vi "Config.vi"(1 "Config_W/R":bool, 2 "Config":T1={"IP"="192.168.0.1", "UserName"="admin", "Password"="admin", "boards_selector_group 1"=0, "boards_selector_group 2"=0, "log_name_group1"="G1", "log_name_group2"="G2", "Port"="COM5", "Delay[s]"=1.0, "on/off"=TRUE, "Graphs_color"=16448250, "Pages_color"=[6901059, 10986955, 11240591, 32639, 32639, 32639, 32639, 16777224, 9868950, 4417895, 8686180, 8686180, 8686180, 8686180], "logs_Path"=path "C:/Users/NEOVP/Documents/HV_DATA"} {"Delay[s]" format="%#_13g"}) -> (0 "Config_read":T1={"IP"="192.168.0.1", "UserName"="admin", "Password"="admin", "boards_selector_group 1"=0, "boards_selector_group 2"=0, "log_name_group1"="G1", "log_name_group2"="G2", "Port"="", "Delay[s]"=1.0, "on/off"=TRUE, "Graphs_color"=16448250, "Pages_color"=[6901059, 10986955, 11240591, 32639, 32639, 32639, 32639, 16777224, 9868950, 4417895, 8686180, 8686180, 8686180, 8686180], "logs_Path"=path ""} {"Delay[s]" format="%#_13g"})   [LabVIEW 2018]
uses:
  <vilib>/Utility/config.llb/Read Key (String).vi
  <vilib>/Utility/config.llb/Read Key (I32).vi
  <vilib>/Utility/config.llb/Read Key (Path).vi
  <vilib>/Utility/config.llb/Read Key (Double).vi
  <vilib>/Utility/config.llb/Read Key (Boolean).vi
  <vilib>/Utility/config.llb/Write Key (String).vi
  <vilib>/Utility/config.llb/Write Key (I32).vi
  <vilib>/Utility/config.llb/Write Key (Path).vi
  <vilib>/Utility/config.llb/Write Key (Double).vi
  <vilib>/Utility/config.llb/Write Key (Boolean).vi
  <vilib>/Utility/config.llb/NI_LVConfig.lvlib
panel:
  in  "Config Template":T1={"IP"="192.168.0.1", "UserName"="admin", "Password"="admin", "boards_selector_group 1"=0, "boards_selector_group 2"=0, "log_name_group1"="G1", "log_name_group2"="G2", "Port"="COM5", "Delay[s]"=1.0, "on/off"=TRUE, "Graphs_color"=16448250, "Pages_color"=[6901059, 10986955, 11240591, 32639, 32639, 32639, 32639, 16777224, 9868950, 4417895, 8686180, 8686180, 8686180, 8686180], "logs_Path"=path "C:/Users/NEOVP/Documents/HV_DATA"} {"Delay[s]" format="%#_13g"}
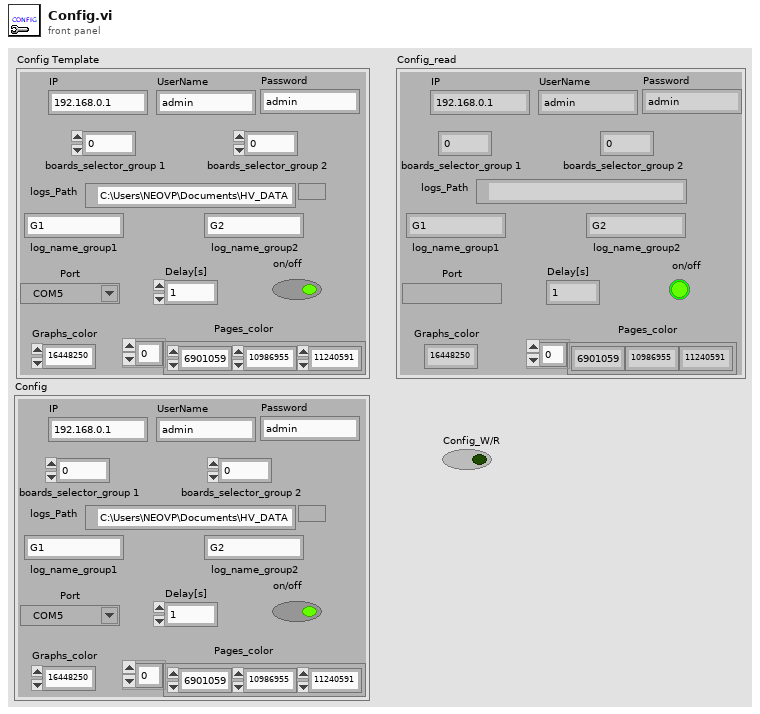
[diagram p1: front panel]
types:
  T1 = cluster{"IP":string, "UserName":string, "Password":string, "boards_selector_group 1":i32, "boards_selector_group 2":i32, "log_name_group1":string, "log_name_group2":string, "Port":refnum<visa-resource-name>, "Delay[s]":dbl, "on/off":bool, "Graphs_color":i32, "Pages_color":i64[], "logs_Path":path}
  T2 = typedef "NI_LVConfig.lvlib/Config Data RefNum.ctl" = refnum<k1>
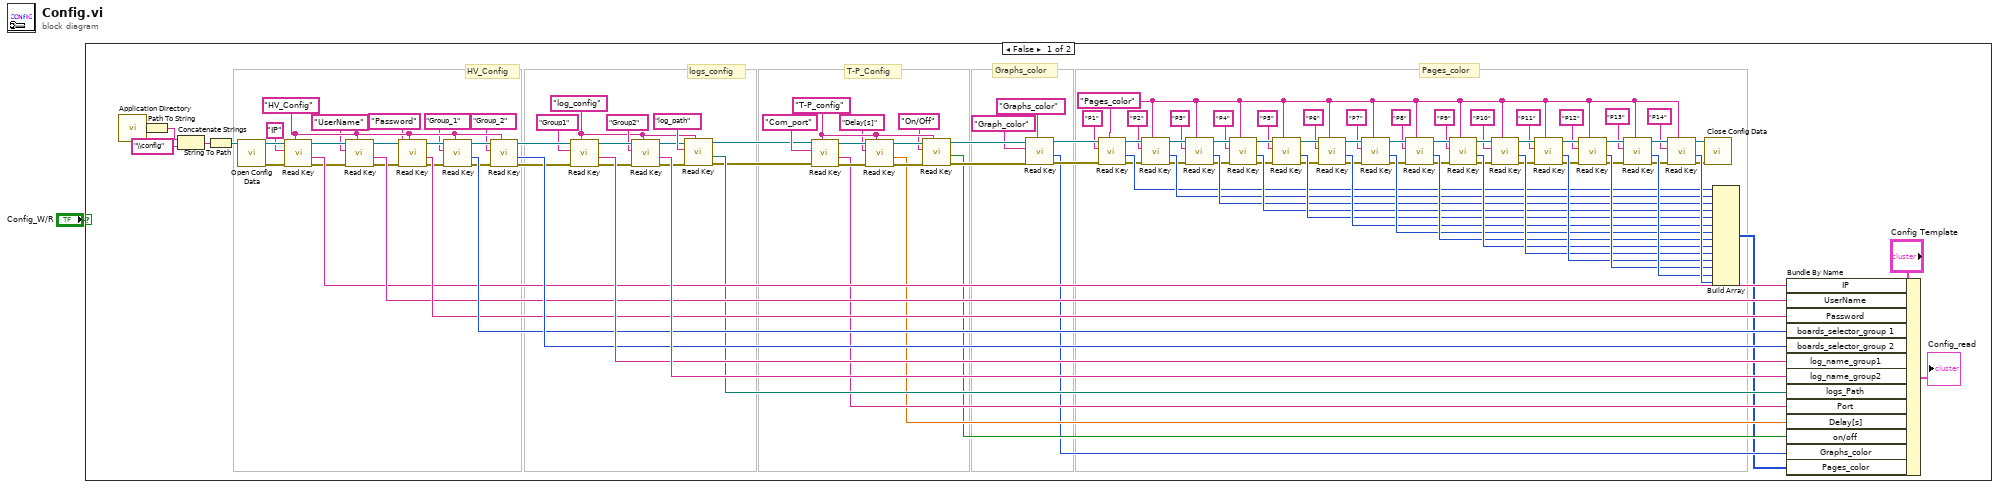
[diagram p0: block diagram]
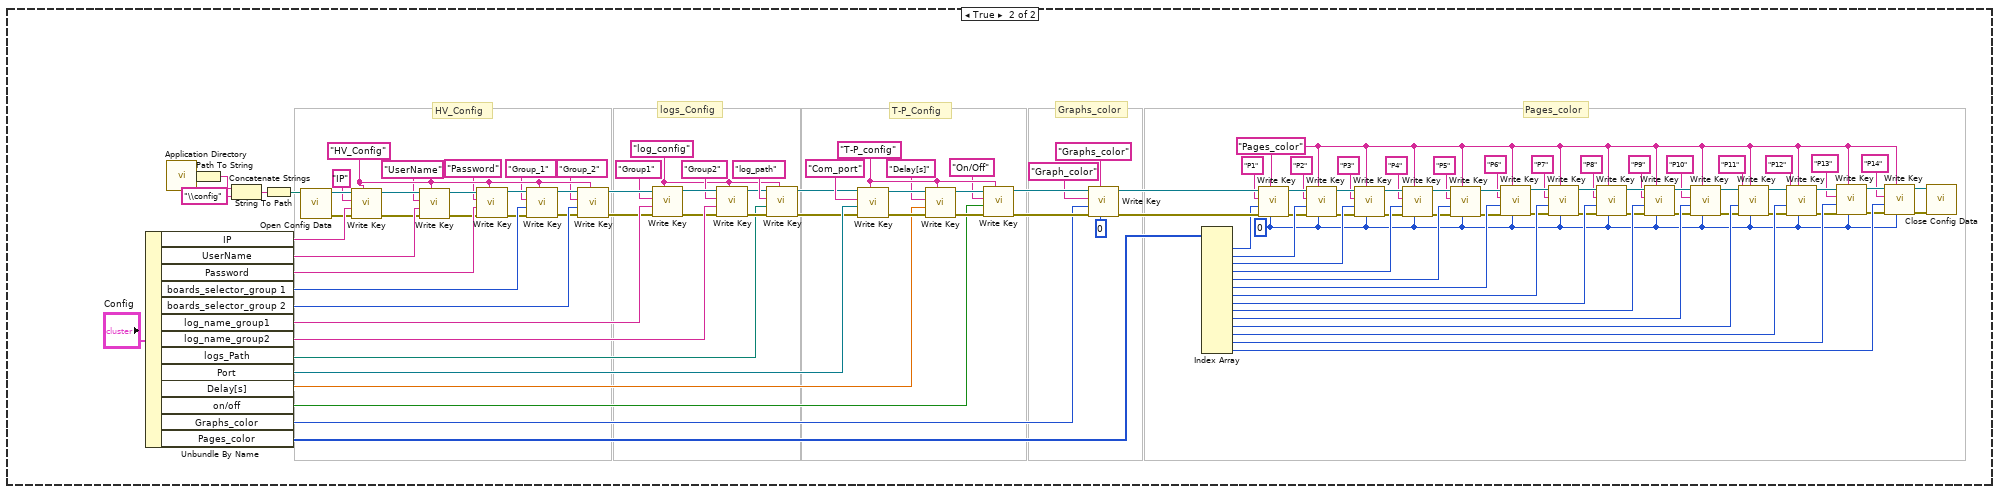
[diagram p2: hidden frame]
diagram:
  n1 = case shown="False" "Config_W/R" {
    frame False {
      w12 = "log_config" ("section")
      w41 = "HV_Config" ("section")
      w35 = "T-P_config" ("section")
      w29 = "Pages_color" ("section")
      # "logs_config"
      # "Pages_color"
      # "Graphs_color"
      # "T-P_Config"
      # "HV_Config"
      n2 = call <vilib>:"Application Directory.vi"() -> ("Application Directory"=w46:path)
      n3 = Path To String(path=w46) -> (string=w45:string)
      n4 = Concatenate Strings(w45, "\\config" ("string")) -> (w44:string)
      n5 = String To Path(string=w44) -> (path=w107:path)
      n6 = call <vilib>:"Open Config Data.vi"("configuration file path"=w107) -> ("error out"=w105:errorcluster, "refnum"=w106:T2)  [unwired: 8 in, 1 out]
      n7 = call-poly <vilib>:"Read Key.vi"("section"=w41, "error in (no error)"=w105, "key"="IP", "refnum"=w106) -> ("error out"=w103:errorcluster, "value"=w110:string, "refnum out"=w104:T2)  [unwired: 4 in, 1 out]
      n8 = call-poly <vilib>:"Read Key.vi"("section"=w41, "error in (no error)"=w103, "key"="UserName", "refnum"=w104) -> ("error out"=w101:errorcluster, "value"=w111:string, "refnum out"=w102:T2)  [unwired: 4 in, 1 out]
      n9 = call-poly <vilib>:"Read Key.vi"("section"=w41, "error in (no error)"=w101, "key"="Password", "refnum"=w102) -> ("error out"=w99:errorcluster, "value"=w112:string, "refnum out"=w100:T2)  [unwired: 4 in, 1 out]
      n10 = call-poly <vilib>:"Read Key.vi"("section"=w41, "error in (no error)"=w99, "key"="Group_1", "refnum"=w100) -> ("error out"=w97:errorcluster, "value"=w113:i32, "refnum out"=w98:T2)  [unwired: 4 in, 1 out]
      n11 = call-poly <vilib>:"Read Key.vi"("section"=w41, "error in (no error)"=w97, "key"="Group_2", "refnum"=w98) -> ("error out"=w93:errorcluster, "value"=w114:i32, "refnum out"=w94:T2)  [unwired: 4 in, 1 out]
      n12 = call-poly <vilib>:"Read Key.vi"("section"=w12, "error in (no error)"=w93, "key"="Group1", "refnum"=w94) -> ("error out"=w96:errorcluster, "value"=w115:string, "refnum out"=w95:T2)  [unwired: 4 in, 1 out]
      n13 = call-poly <vilib>:"Read Key.vi"("section"=w12, "error in (no error)"=w96, "key"="Group2", "refnum"=w95) -> ("error out"=w3:errorcluster, "value"=w116:string, "refnum out"=w5:T2)  [unwired: 4 in, 1 out]
      n14 = call-poly <vilib>:"Read Key.vi"("section"=w12, "error in (no error)"=w3, "key"="log_path", "refnum"=w5) -> ("error out"=w2:errorcluster, "value"=w11:path, "refnum out"=w4:T2)  [unwired: 4 in, 1 out]
      n15 = call-poly <vilib>:"Read Key.vi"("section"=w35, "error in (no error)"=w2, "key"="Com_port", "refnum"=w4) -> ("error out"=w90:errorcluster, "value"=w10:string, "refnum out"=w89:T2)  [unwired: 4 in, 1 out]
      n16 = call-poly <vilib>:"Read Key.vi"("section"=w35, "error in (no error)"=w90, "key"="Delay[s]", "refnum"=w89) -> ("error out"=w92:errorcluster, "value"=w9:dbl, "refnum out"=w91:T2)  [unwired: 4 in, 1 out]
      n17 = call-poly <vilib>:"Read Key.vi"("section"=w35, "error in (no error)"=w92, "key"="On/Off", "refnum"=w91) -> ("error out"=w118:errorcluster, "value"=w8:bool, "refnum out"=w117:T2)  [unwired: 4 in, 1 out]
      n18 = call-poly <vilib>:"Read Key.vi"("section"="Graphs_color", "error in (no error)"=w118, "key"="Graph_color", "refnum"=w117) -> ("error out"=w120:errorcluster, "value"=w7:i32, "refnum out"=w119:T2)  [unwired: 4 in, 1 out]
      n19 = call-poly <vilib>:"Read Key.vi"("section"=w29, "error in (no error)"=w120, "key"="P1", "refnum"=w119) -> ("error out"=w70:errorcluster, "value"=w74:i32, "refnum out"=w71:T2)  [unwired: 4 in, 1 out]
      n20 = call-poly <vilib>:"Read Key.vi"("section"=w29, "error in (no error)"=w70, "key"="P2", "refnum"=w71) -> ("error out"=w68:errorcluster, "value"=w75:i32, "refnum out"=w69:T2)  [unwired: 4 in, 1 out]
      n21 = call-poly <vilib>:"Read Key.vi"("section"=w29, "error in (no error)"=w68, "key"="P3", "refnum"=w69) -> ("error out"=w66:errorcluster, "value"=w76:i32, "refnum out"=w67:T2)  [unwired: 4 in, 1 out]
      n22 = call-poly <vilib>:"Read Key.vi"("section"=w29, "error in (no error)"=w66, "key"="P4", "refnum"=w67) -> ("error out"=w73:errorcluster, "value"=w77:i32, "refnum out"=w72:T2)  [unwired: 4 in, 1 out]
      n23 = call-poly <vilib>:"Read Key.vi"("section"=w29, "error in (no error)"=w73, "key"="P5", "refnum"=w72) -> ("error out"=w60:errorcluster, "value"=w78:i32, "refnum out"=w59:T2)  [unwired: 4 in, 1 out]
      n24 = call-poly <vilib>:"Read Key.vi"("section"=w29, "error in (no error)"=w60, "key"="P6", "refnum"=w59) -> ("error out"=w64:errorcluster, "value"=w79:i32, "refnum out"=w63:T2)  [unwired: 4 in, 1 out]
      n25 = call-poly <vilib>:"Read Key.vi"("section"=w29, "error in (no error)"=w64, "key"="P7", "refnum"=w63) -> ("error out"=w80:errorcluster, "value"=w81:i32, "refnum out"=w65:T2)  [unwired: 4 in, 1 out]
      n26 = call-poly <vilib>:"Read Key.vi"("section"=w29, "error in (no error)"=w80, "key"="P8", "refnum"=w65) -> ("error out"=w61:errorcluster, "value"=w82:i32, "refnum out"=w62:T2)  [unwired: 4 in, 1 out]
      n27 = call-poly <vilib>:"Read Key.vi"("section"=w29, "error in (no error)"=w61, "key"="P9", "refnum"=w62) -> ("error out"=w50:errorcluster, "value"=w83:i32, "refnum out"=w49:T2)  [unwired: 4 in, 1 out]
      n28 = call-poly <vilib>:"Read Key.vi"("section"=w29, "error in (no error)"=w50, "key"="P10", "refnum"=w49) -> ("error out"=w54:errorcluster, "value"=w84:i32, "refnum out"=w53:T2)  [unwired: 4 in, 1 out]
      n29 = call-poly <vilib>:"Read Key.vi"("section"=w29, "error in (no error)"=w54, "key"="P11", "refnum"=w53) -> ("error out"=w51:errorcluster, "value"=w85:i32, "refnum out"=w52:T2)  [unwired: 4 in, 1 out]
      n30 = call-poly <vilib>:"Read Key.vi"("section"=w29, "error in (no error)"=w51, "key"="P12", "refnum"=w52) -> ("error out"=w57:errorcluster, "value"=w86:i32, "refnum out"=w58:T2)  [unwired: 4 in, 1 out]
      n31 = call-poly <vilib>:"Read Key.vi"("section"=w29, "error in (no error)"=w57, "key"="P13", "refnum"=w58) -> ("error out"=w55:errorcluster, "value"=w87:i32, "refnum out"=w56:T2)  [unwired: 4 in, 1 out]
      n32 = call-poly <vilib>:"Read Key.vi"("section"=w29, "error in (no error)"=w55, "key"="P14", "refnum"=w56) -> ("error out"=w47:errorcluster, "value"=w88:i32, "refnum out"=w48:T2)  [unwired: 4 in, 1 out]
      n33 = call <vilib>:"Close Config Data.vi"("error in (no error)"=w47, "refnum"=w48) -> ()  [unwired: 8 in, 2 out]
      n34 = Build Array(w74, w75, w76, w77, w78, w79, w81, w82, w83, w84, w85, w86, w87, w88) -> (w6:i32[])
      n35 = Bundle By Name(cluster="Config Template", "IP"=w110, "UserName"=w111, "Password"=w112, "boards_selector_group 1"=w113, "boards_selector_group 2"=w114, "log_name_group1"=w115, "log_name_group2"=w116, "logs_Path"=w11, "Port"=w10, "Delay[s]"=w9, "on/off"=w8, "Graphs_color"=w7, "Pages_color"=w6) -> (→"Config_read":T1)
    }
    frame True {
      w164 = "T-P_config" ("section")
      w157 = i16 0 ("precision (6)")
      w156 = "Pages_color" ("section")
      w121 = "log_config" ("section")
      w139 = "HV_Config" ("section")
      # "logs_Config"
      # "Pages_color"
      # "Graphs_color"
      # "T-P_Config"
      # "HV_Config"
      n36 = Unbundle By Name("Config") -> ("IP"=w234:string, "UserName"=w235:string, "Password"=w236:string, "boards_selector_group 1"=w237:i32, "boards_selector_group 2"=w238:i32, "log_name_group1"=w239:string, "log_name_group2"=w240:string, "logs_Path"=w128:path, "Port"=w127:refnum<visa-resource-name>, "Delay[s]"=w126:dbl, "on/off"=w125:bool, "Graphs_color"=w124:i32, "Pages_color"=w123:i64[])
      n37 = call <vilib>:"Application Directory.vi"() -> ("Application Directory"=w167:path)
      n38 = Path To String(path=w167) -> (string=w166:string)
      n39 = Concatenate Strings(w166, "\\config" ("string")) -> (w165:string)
      n40 = String To Path(string=w165) -> (path=w228:path)
      n41 = call <vilib>:"Open Config Data.vi"("configuration file path"=w228) -> ("error out"=w169:errorcluster, "refnum"=w168:T2)  [unwired: 8 in, 1 out]
      n42 = call-poly <vilib>:"Write Key.vi"("section"=w139, "error in (no error)"=w169, "value"=w234, "key"="IP", "refnum"=w168) -> ("error out"=w171:errorcluster, "refnum out"=w170:T2)  [unwired: 4 in, 1 out]
      n43 = call-poly <vilib>:"Write Key.vi"("section"=w139, "error in (no error)"=w171, "value"=w235, "key"="UserName", "refnum"=w170) -> ("error out"=w173:errorcluster, "refnum out"=w172:T2)  [unwired: 4 in, 1 out]
      n44 = call-poly <vilib>:"Write Key.vi"("section"=w139, "error in (no error)"=w173, "value"=w236, "key"="Password", "refnum"=w172) -> ("error out"=w175:errorcluster, "refnum out"=w174:T2)  [unwired: 4 in, 1 out]
      n45 = call-poly <vilib>:"Write Key.vi"("section"=w139, "error in (no error)"=w175, "value"=w237, "key"="Group_1", "refnum"=w174) -> ("error out"=w177:errorcluster, "refnum out"=w176:T2)  [unwired: 4 in, 1 out]
      n46 = call-poly <vilib>:"Write Key.vi"("section"=w139, "error in (no error)"=w177, "value"=w238, "key"="Group_2", "refnum"=w176) -> ("error out"=w181:errorcluster, "refnum out"=w180:T2)  [unwired: 4 in, 1 out]
      n47 = call-poly <vilib>:"Write Key.vi"("section"=w121, "error in (no error)"=w181, "value"=w239, "key"="Group1", "refnum"=w180) -> ("error out"=w178:errorcluster, "refnum out"=w179:T2)  [unwired: 4 in, 1 out]
      n48 = call-poly <vilib>:"Write Key.vi"("section"=w121, "error in (no error)"=w178, "value"=w240, "key"="Group2", "refnum"=w179) -> ("error out"=w130:errorcluster, "refnum out"=w131:T2)  [unwired: 4 in, 1 out]
      n49 = call-poly <vilib>:"Write Key.vi"("section"=w121, "error in (no error)"=w130, "value"=w128, "key"="log_path", "refnum"=w131) -> ("error out"=w122:errorcluster, "refnum out"=w129:T2)  [unwired: 4 in, 1 out]
      n50 = call-poly <vilib>:"Write Key.vi"("section"=w164, "error in (no error)"=w122, "value"=w127, "key"="Com_port", "refnum"=w129) -> ("error out"=w226:errorcluster, "refnum out"=w227:T2)  [unwired: 4 in, 1 out]
      n51 = call-poly <vilib>:"Write Key.vi"("section"=w164, "error in (no error)"=w226, "value"=w126, "key"="Delay[s]", "refnum"=w227) -> ("error out"=w224:errorcluster, "refnum out"=w225:T2)  [unwired: 4 in, 1 out]
      n52 = call-poly <vilib>:"Write Key.vi"("section"=w164, "error in (no error)"=w224, "value"=w125, "key"="On/Off", "refnum"=w225) -> ("error out"=w230:errorcluster, "refnum out"=w229:T2)  [unwired: 4 in, 1 out]
      n53 = call-poly <vilib>:"Write Key.vi"("precision (6)"=i16 0, "section"="Graphs_color", "error in (no error)"=w230, "value"=w124, "key"="Graph_color", "refnum"=w229) -> ("error out"=w231:errorcluster, "refnum out"=w232:T2)  [unwired: 3 in, 1 out]
      n54 = Index Array(array=w123) -> (element #1=w210:i64, element #2=w211:i64, element #3=w212:i64, element #4=w213:i64, element #5=w214:i64, element #6=w215:i64, element #7=w216:i64, element #8=w217:i64, element #9=w218:i64, element #10=w219:i64, element #11=w220:i64, element #12=w221:i64, element #13=w222:i64, element #14=w223:i64)  [unwired: 14 in]
      n55 = call-poly <vilib>:"Write Key.vi"("precision (6)"=w157, "section"=w156, "error in (no error)"=w231, "value"=w210, "key"="P1", "refnum"=w232) -> ("error out"=w185:errorcluster, "refnum out"=w184:T2)  [unwired: 3 in, 1 out]
      n56 = call-poly <vilib>:"Write Key.vi"("precision (6)"=w157, "section"=w156, "error in (no error)"=w185, "value"=w211, "key"="P2", "refnum"=w184) -> ("error out"=w187:errorcluster, "refnum out"=w186:T2)  [unwired: 3 in, 1 out]
      n57 = call-poly <vilib>:"Write Key.vi"("precision (6)"=w157, "section"=w156, "error in (no error)"=w187, "value"=w212, "key"="P3", "refnum"=w186) -> ("error out"=w189:errorcluster, "refnum out"=w188:T2)  [unwired: 3 in, 1 out]
      n58 = call-poly <vilib>:"Write Key.vi"("precision (6)"=w157, "section"=w156, "error in (no error)"=w189, "value"=w213, "key"="P4", "refnum"=w188) -> ("error out"=w182:errorcluster, "refnum out"=w183:T2)  [unwired: 3 in, 1 out]
      n59 = call-poly <vilib>:"Write Key.vi"("precision (6)"=w157, "section"=w156, "error in (no error)"=w182, "value"=w214, "key"="P5", "refnum"=w183) -> ("error out"=w196:errorcluster, "refnum out"=w197:T2)  [unwired: 3 in, 1 out]
      n60 = call-poly <vilib>:"Write Key.vi"("precision (6)"=w157, "section"=w156, "error in (no error)"=w196, "value"=w215, "key"="P6", "refnum"=w197) -> ("error out"=w192:errorcluster, "refnum out"=w193:T2)  [unwired: 3 in, 1 out]
      n61 = call-poly <vilib>:"Write Key.vi"("precision (6)"=w157, "section"=w156, "error in (no error)"=w192, "value"=w216, "key"="P7", "refnum"=w193) -> ("error out"=w190:errorcluster, "refnum out"=w191:T2)  [unwired: 3 in, 1 out]
      n62 = call-poly <vilib>:"Write Key.vi"("precision (6)"=w157, "section"=w156, "error in (no error)"=w190, "value"=w217, "key"="P8", "refnum"=w191) -> ("error out"=w195:errorcluster, "refnum out"=w194:T2)  [unwired: 3 in, 1 out]
      n63 = call-poly <vilib>:"Write Key.vi"("precision (6)"=w157, "section"=w156, "error in (no error)"=w195, "value"=w218, "key"="P9", "refnum"=w194) -> ("error out"=w206:errorcluster, "refnum out"=w207:T2)  [unwired: 3 in, 1 out]
      n64 = call-poly <vilib>:"Write Key.vi"("precision (6)"=w157, "section"=w156, "error in (no error)"=w206, "value"=w219, "key"="P10", "refnum"=w207) -> ("error out"=w202:errorcluster, "refnum out"=w203:T2)  [unwired: 3 in, 1 out]
      n65 = call-poly <vilib>:"Write Key.vi"("precision (6)"=w157, "section"=w156, "error in (no error)"=w202, "value"=w220, "key"="P11", "refnum"=w203) -> ("error out"=w205:errorcluster, "refnum out"=w204:T2)  [unwired: 3 in, 1 out]
      n66 = call-poly <vilib>:"Write Key.vi"("precision (6)"=w157, "section"=w156, "error in (no error)"=w205, "value"=w221, "key"="P12", "refnum"=w204) -> ("error out"=w199:errorcluster, "refnum out"=w198:T2)  [unwired: 3 in, 1 out]
      n67 = call-poly <vilib>:"Write Key.vi"("precision (6)"=w157, "section"=w156, "error in (no error)"=w199, "value"=w222, "key"="P13", "refnum"=w198) -> ("error out"=w201:errorcluster, "refnum out"=w200:T2)  [unwired: 3 in, 1 out]
      n68 = call-poly <vilib>:"Write Key.vi"("precision (6)"=w157, "section"=w156, "error in (no error)"=w201, "value"=w223, "key"="P14", "refnum"=w200) -> ("error out"=w209:errorcluster, "refnum out"=w208:T2)  [unwired: 3 in, 1 out]
      n69 = call <vilib>:"Close Config Data.vi"("error in (no error)"=w209, "refnum"=w208) -> ()  [unwired: 8 in, 2 out]
    }
  }
